vi "test 05 - New Chan with no loss.vi"() -> ()   [LabVIEW 2020]
uses:
  UI_Actor/UI_Actor/ctl_AR_Parameters.ctl
  UI_Actor/UI_Actor/ctl_AR_Mode.ctl
  support/Databox.lvlibp/TypesTools/Config/Config.lvclass
  support/Databox.lvlibp/TypesTools/Data/Data.lvclass
  support/Databox.lvlibp/TypesTools/Data/TypeEnum.ctl
  UIA_UTsupport/UIA_UTsupport.lvclass
  D:/Projets/STEP AT/UI Actor/UI_Actor/UI_Actor/UI_Actor.lvclass
  UI_Actor/UI_Actor Messages/UI_AutoRefresh Msg/UI_AutoRefresh Msg.lvclass/UI_AutoRefresh Msg.ctl
  f7e9fdf2-272c-4cde-b3ea-907668245b3f.vi
  e3e33372-f0f8-45c8-a109-52282a8919ad.vi
  UIA_UTsupport/gloglo.vi
  support/Actor Framework.lvlibp/1abvi3w/vi.lib/ActorFramework/Message Enqueuer/Enqueue.vi
  UI_Actor/UI_Actor Messages/UI_AutoRefresh Msg/UI_AutoRefresh Msg.lvclass
  UI_Actor/UI_Actor/UI_Actor.lvclass
  support/Actor Framework.lvlibp/1abvi3w/vi.lib/ActorFramework/Stop Msg/Stop Msg.lvclass
panel:
  out "PASS":bool
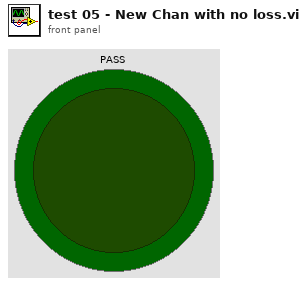
[diagram p1: front panel]
types:
  T1 = typedef "Databox.lvlibp/Data.lvclass/TypeEnum.ctl" = enum16{"Boolean", "SByte", "Byte", "Int16", "UInt16", "Int32", "UInt32", "Int64", "UInt64", "Float", "Double", "String", "DateTime", "ByteString", "Array of Boolean", "Array of SByte", "Array of Byte", "Array of Int16", "Array of UInt16", "Array of Int32", "Array of UInt32", "Array of Int64", "Array of UInt64", "Array of Float", "Array of Double", "Array of String", "Array of DateTime", "Array of ByteString", "Matrix of Boolean", "Matrix of SByte", "Matrix of Byte", "Matrix of Int16", "Matrix of UInt16", "Matrix of Int32", "Matrix of UInt32", "Matrix of Int64", "Matrix of UInt64", "Matrix of Float", "Matrix of Double", "Matrix of String ", "Matrix of DateTime", "Matrix of ByteString"}
  T2 = cluster{"Ch.Conf":refnum<class "Config.lvclass">, "Data":refnum<class "Data.lvclass">[]}
  T3 = typedef "UI_Actor.lvlib/UI_Actor.lvclass/ctl_AR_Parameters.ctl" = cluster{"Write TipStrips with details (T)":bool, "Write Captions with UserLabels (T)":bool, "Mode (ind only)":T4, "Enable nested stream (T)":bool}
  T4 = typedef "UI_Actor.lvlib/UI_Actor.lvclass/ctl_AR_Mode.ctl" = enum16{"Controls only", "Indicators only", "All"}
  T5 = cluster{"Ch.Conf":refnum<class "Config.lvclass">, "Data":refnum<class "Data.lvclass">[]}[]
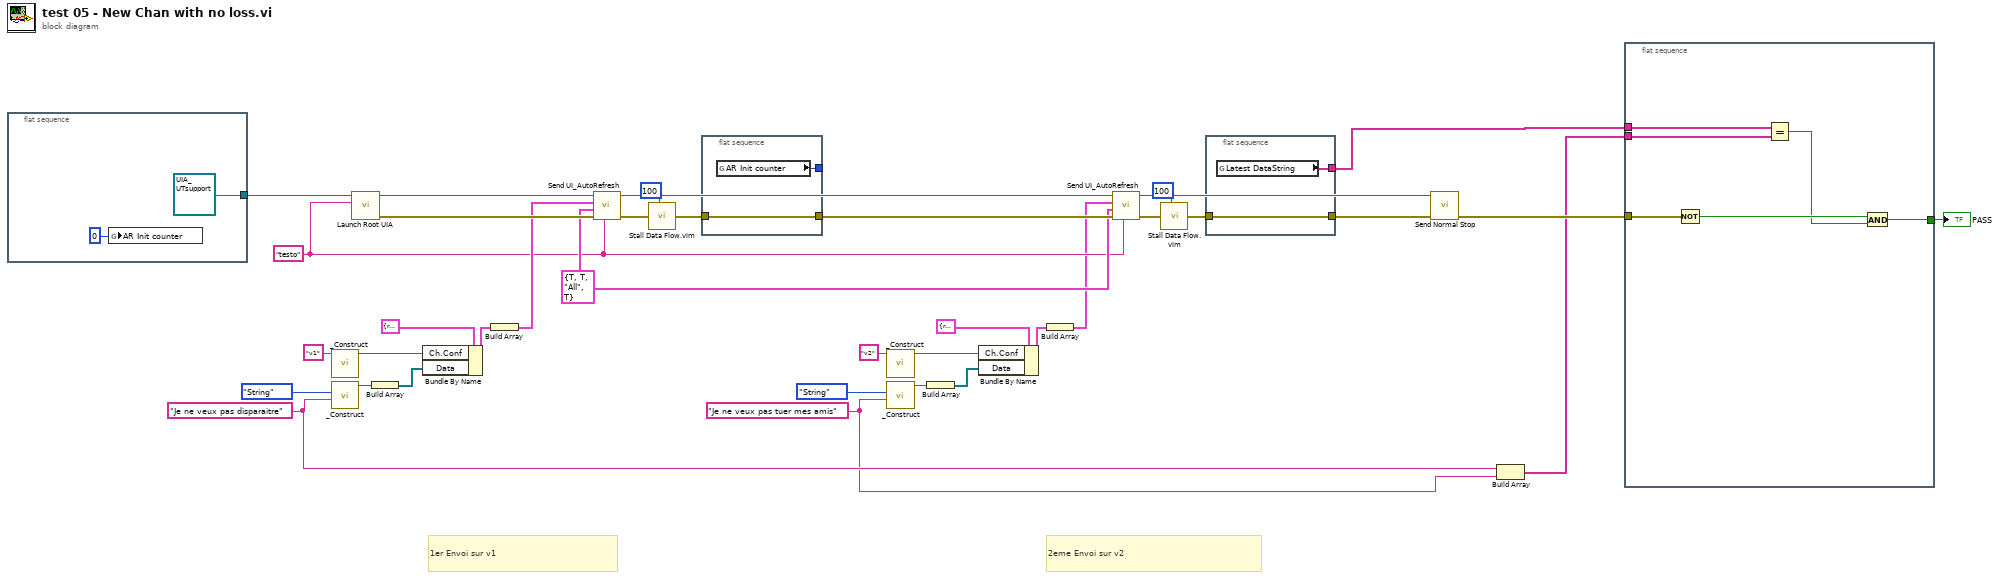
[diagram p0: block diagram]
diagram:
  w3 = "Je ne veux pas tuer mes amis" ("System Label")
  w4 = "Je ne veux pas disparaitre" ("System Label")
  w16 = "testo" ("Actor Name")
  w17 = T3 {"Write TipStrips with details (T)"=TRUE, "Write Captions with UserLabels (T)"=TRUE, "Mode (ind only)"=enum."All", "Enable nested stream (T)"=TRUE} ("Parameters (Tipstrips,Captions,All)")
  # "2eme Envoi sur v2"
  # "1er Envoi sur v1"
  n1 = flat-sequence {
    tunnel: [refnum<class "UIA_UTsupport.lvclass"> refnum ("UIA_UTsupport.lvlib:UIA_UTsupport.lvclass")] -> w26
    frame #0 {
      n2 = global write "gloglo.vi" "AR Init counter"(0 ("AR Init counter")) -> ()
    }
  }
  n3 = call "_Construct.vi"("System Label"="v1") -> ("Ch.Conf out"=w36:refnum<class "Config.lvclass">)  [unwired: 13 in, 1 out]
  n4 = call "_Construct.vi"("Value"=w4, "Type"=TypeEnum."String") -> ("Ch.TData out"=w35:refnum<class "Data.lvclass">)  [unwired: 8 in, 1 out]
  n5 = call "Launch Root UIA.vi"("Actor Name"=w16, "UI_Actor in"=w26) -> ("error out"=w37:errorcluster, "Actor's Enqueuer"=w32:refnum<class "Message Enqueuer.lvclass">)  [unwired: 8 in]
  n6 = Build Array(w35) -> (w34:refnum<class "Data.lvclass">[])
  n7 = Bundle By Name(cluster=T2 {"Ch.Conf"=refnum, "Data"=[]} ("Cluster"), "Ch.Conf"=w36, "Data"=w34) -> (w18:T2)
  n8 = Build Array(w18) -> (w25:T5)
  n9 = call "Send UI_AutoRefresh.vi"("Sourcer name"=w16, "error in (no error)"=w37, "Parameters (Tipstrips,Captions,All)"=w17, "Data chunk"=w25, "Message Enqueuer"=w32) -> ("error out"=w24:errorcluster, "Message Enqueuer out"=w29:refnum<class "Message Enqueuer.lvclass">)  [unwired: 5 in]
  n10 = call "Stall Data Flow.vim"("value in"=w24, "milliseconds to wait"=u32 100) -> ("value out"=w21:errorcluster)  [unwired: 1 out]
  n11 = flat-sequence {
    tunnel: [w41] -> w22
    tunnel: w21 -> [w41]
    tunnel: [w40] -> _
    frame #0 {
      n12 = global read "gloglo.vi" "AR Init counter"() -> (w40:i32)
    }
  }
  n13 = call "_Construct.vi"("System Label"="v2") -> ("Ch.Conf out"=w6:refnum<class "Config.lvclass">)  [unwired: 13 in, 1 out]
  n14 = call "_Construct.vi"("Value"=w3, "Type"=TypeEnum."String") -> ("Ch.TData out"=w7:refnum<class "Data.lvclass">)  [unwired: 8 in, 1 out]
  n15 = Build Array(w7) -> (w8:refnum<class "Data.lvclass">[])
  n16 = Bundle By Name(cluster=T2 {"Ch.Conf"=refnum, "Data"=[]} ("Cluster"), "Ch.Conf"=w6, "Data"=w8) -> (w12:T2)
  n17 = Build Array(w12) -> (w5:T5)
  n18 = call "Send UI_AutoRefresh.vi"("Sourcer name"=w16, "error in (no error)"=w22, "Parameters (Tipstrips,Captions,All)"=w17, "Data chunk"=w5, "Message Enqueuer"=w29) -> ("error out"=w14:errorcluster, "Message Enqueuer out"=w20:refnum<class "Message Enqueuer.lvclass">)  [unwired: 5 in]
  n19 = call "Stall Data Flow.vim"("value in"=w14, "milliseconds to wait"=u32 100) -> ("value out"=w13:errorcluster)  [unwired: 1 out]
  n20 = flat-sequence {
    tunnel: [w43] -> w19
    tunnel: w13 -> [w43]
    tunnel: [w42] -> w1
    frame #0 {
      n21 = global read "gloglo.vi" "Latest DataString"() -> (w42:string[])
    }
  }
  n22 = call "Send Normal Stop.vi"("error in (no error)"=w19, "Message Enqueuer"=w20) -> ("error out"=w30:errorcluster)  [unwired: 9 in]
  n23 = Build Array(w4, w3) -> (w2:string[])
  n24 = flat-sequence {
    tunnel: w30 -> [w49]
    tunnel: [w47] -> w31
    tunnel: w2 -> [w45]
    tunnel: w1 -> [w44]
    frame #0 {
      n25 = Not(x=w49) -> (.not. x?=w48:bool)
      n26 = Equal?(x=w44, y=w45) -> (x = y?=w46:bool)
      n27 = And(x=w48, y=w46) -> (x .and. y?=w47:bool)
    }
  }
  "PASS" <- w31
